vi "Create LVLIB Copies and Replace in LVPROJ.vi"(6 "copy":T1(ring), 7 "template base name":string, 8 "error in":errorcluster, 9 "CD name":string, 10 "relative path of LVLIB folders":path[](array[path]), 11 "custom device path":path) -> (0 "error out":errorcluster, 3 "custom device path out":path)   [LabVIEW 2020, in "Template Tool.lvlib"]
uses:
  Template Tool.lvlib
panel:
  out "relinked subVIs":string[](array[string])
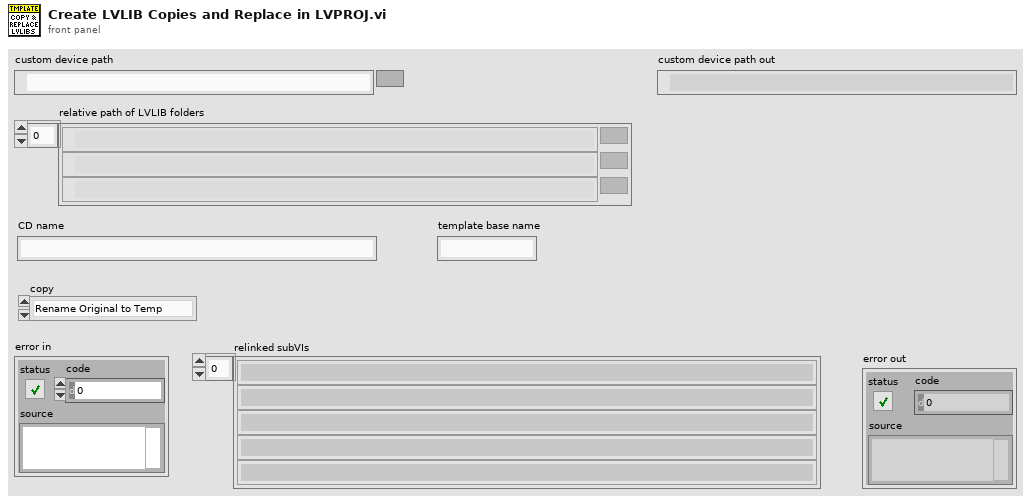
[diagram p1: front panel]
types:
  T1 = enum16{"Rename Original to Temp", "Rename Temp to Original"}
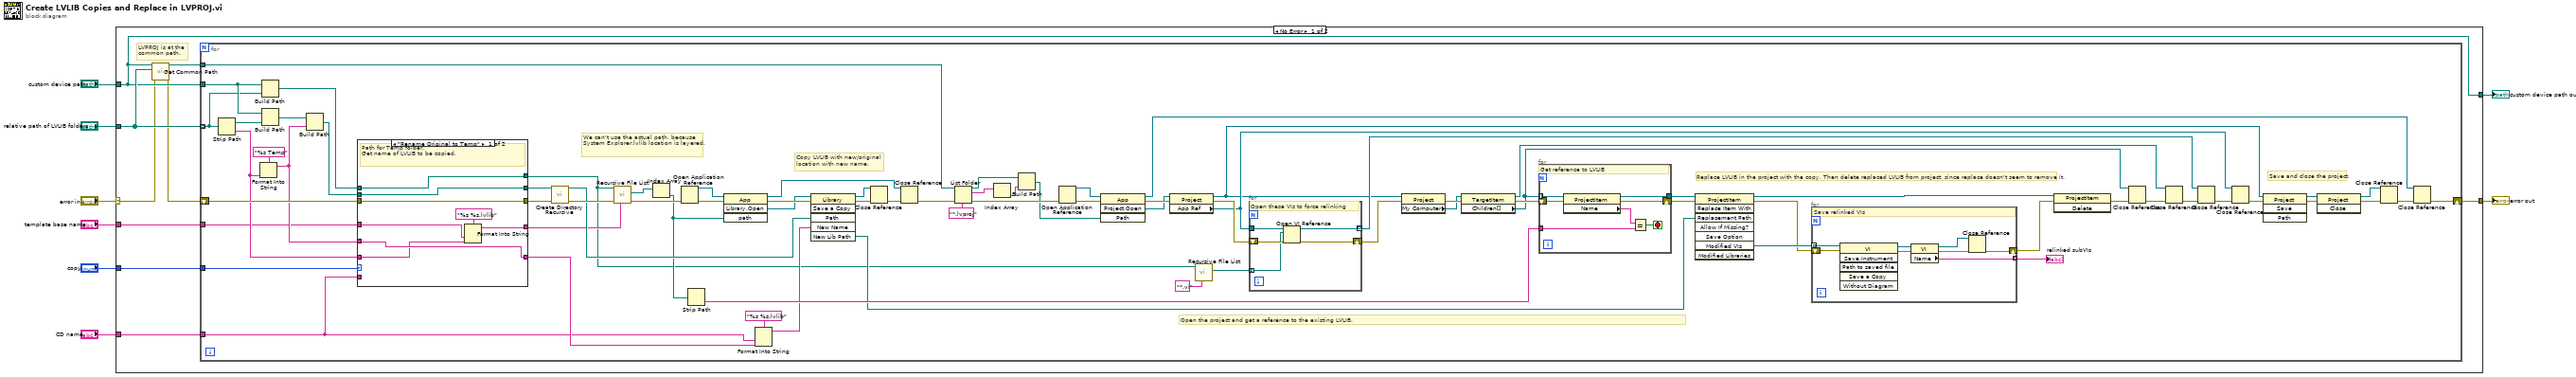
[diagram p0: block diagram]
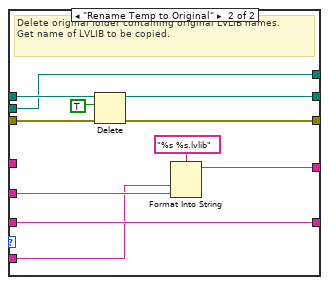
[diagram p2: hidden frame]
diagram:
  n1 = case shown="No Error" "error in" {
    selector: "error in" -> [w13 w136]
    tunnel: "custom device path" -> [w15 w135]
    tunnel: [w17 w136] -> w7
    tunnel: [w15 w135] -> w6
    tunnel: "relative path of LVLIB folders" -> [w16 _]
    tunnel: "copy" -> [w11 _]
    tunnel: "CD name" -> [w10 _]
    tunnel: "template base name" -> [w9 _]
    frame No Error {
      # "LVPROJ is at the common path."
      n2 = call "Get Common Path.vi"("error in"=w13, "relative path of LVLIB folders"=w16, "custom device path"=w15) -> ("error out"=w12:errorcluster, "common path"=w14:path)  [unwired: 7 in]
      n3 = for {
        tunnel: w15 -> [w66]
        tunnel: w16 -> [w65] mode=indexing
        shift-right: [w56] -> w17
        shift-left: w12 -> [w42]
        tunnel: w14 -> [w37]
        tunnel: w11 -> [w22]
        tunnel: w10 -> [w19]
        tunnel: w9 -> [w18]
        # "We can't use the actual path, because System Explorer.lvlib location is layered."
        # "Save and close the project."
        # "Replace LVLIB in the project with the copy. Then delete replaced LVLIB from project, since replace doesn't seem to remove it."
        # "Open the project and get a reference to the existing LVLIB."
        # "Copy LVLIB with new/original location with new name."
        n4 = Strip Path(path=w65) -> (stripped path=w67:path, name=w24:string)
        n5 = Format Into String(format string="%s Temp" ("string"), w24) -> (resulting string=w31:string)  [unwired: 2 in, 1 out]
        n6 = Build Path(base path=w66, name or relative path=w65) -> (appended path=w40:path)
        n7 = Build Path(base path=w66, name or relative path=w67) -> (appended path=w38:path)
        n8 = Build Path(base path=w38, name or relative path=w31) -> (appended path=w21:path)
        n9 = case shown="\"Rename Original to Temp\"" w22 {
          tunnel: w42 -> [w123 w133]
          tunnel: [w123 w132] -> w41
          tunnel: w40 -> [w118 w131]
          tunnel: [w122 w130] -> w39
          tunnel: [w120 w128] -> w36
          tunnel: w31 -> [w119 w127]
          tunnel: w24 -> [w117 w126]
          tunnel: [w119 w126] -> w23
          tunnel: w21 -> [w122 w125]
          tunnel: [w118 w125] -> w20
          tunnel: w19 -> [_ w124]
          tunnel: w18 -> [w116 _]
          frame "Rename Original to Temp" {
            # "Path for Temp folder.\nGet name of LVLIB to be copied."
            n10 = Format Into String(format string="%s %s.lvlib" ("pattern"), w116, w117) -> (resulting string=w120:string)  [unwired: 2 in, 1 out]
          }
          frame "Rename Temp to Original" {
            # "Delete original folder containing original LVLIB names.\nGet name of LVLIB to be copied."
            n11 = Delete(path (use dialog)=w131, entire hierarchy (F)=TRUE, error in=w133) -> (deleted path=w130:path, error out=w132:errorcluster)  [unwired: 2 in, 1 out]
            n12 = Format Into String(format string="%s %s.lvlib" ("pattern"), w124, w127) -> (resulting string=w128:string)  [unwired: 2 in, 1 out]
          }
        }
        n13 = call <vilib>:"Create Directory Recursive.vi"("error in (no error)"=w41, "directory"=w39) -> ("error out"=w87:errorcluster, "directory copy"=w53:path)  [unwired: 3 in, 1 out]
        n14 = call <vilib>:"Recursive File List.vi"("pattern"=w36, "error in (no error)"=w87, "Folder Path"=w20) -> ("error out"=w86:errorcluster, "All Files in Dir"=w95:path[])  [unwired: 4 in, 3 out]
        n15 = Index Array(array=w95) -> (element=w35:path)  [unwired: 1 in]
        n16 = Open Application Reference(8:w86) -> (0:w85:errorcluster, 3:w94:refnum<vi>)  [unwired: 3 in]
        n17 = Strip Path(path=w35) -> (name=w34:string)  [unwired: 1 out]
        n18 = invoke class="App" method="Library.Open"(reference=w94, error in=w85, "path"=w35) -> (reference out=w93:refnum<vi>, error out=w91:errorcluster, "Open Library"=w88:refnum<vi>)  [unwired: 1 in, 1 out]
        n19 = Format Into String(format string="%s %s.lvlib" ("y"), w19, w23) -> (resulting string=w29:string)  [unwired: 2 in, 1 out]
        n20 = invoke class="Library" method="Save a Copy"(reference=w88, error in=w91, "Path"=w53, "New Name"=w29) -> (reference out=w90:refnum<vi>, error out=w89:errorcluster, "New Lib Path"=w33:path)  [unwired: 2 in, 3 out]
        n21 = Close Reference(reference=w90, error in (no error)=w89) -> (error out=w92:errorcluster)
        n22 = Close Reference(reference=w93, error in (no error)=w92) -> (error out=w68:errorcluster)
        n23 = List Folder(path=w37, pattern="*.lvproj", error in=w68) -> (path out=w80:path, filenames=w79:string[], error out=w83:errorcluster)  [unwired: 1 in, 1 out]
        n24 = Index Array(array=w79) -> (element=w81:string)  [unwired: 1 in]
        n25 = Build Path(base path=w80, name or relative path=w81) -> (appended path=w64:path)
        n26 = Open Application Reference(8:w83) -> (0:w84:errorcluster, 3:w82:refnum<vi>)  [unwired: 3 in]
        n27 = invoke class="App" method="Project.Open"(reference=w82, error in=w84, "Path"=w64) -> (reference out=w71:refnum<vi>, error out=w62:errorcluster, "Project:Open"=w60:refnum<vi>)  [unwired: 1 in, 1 out]
        n28 = property class="Project"(reference=w60, error in=w62) -> (reference out=w28:refnum<vi>, error out=w63:errorcluster, "App Ref"=w58:refnum<vi>)
        n29 = call <vilib>:"Recursive File List.vi"("pattern"="*.vi", "Folder Path"=w20) -> ("All Files in Dir"=w43:path[])  [unwired: 5 in, 4 out]
        n30 = for {
          tunnel: w58 -> [w115]
          tunnel: [w112] -> w57 mode=indexing
          tunnel: w43 -> [w113] mode=indexing
          shift-right: [w111] -> w61
          shift-left: w63 -> [w114]
          # "Open these VIs to force relinking"
          n31 = Open VI Reference(application reference (local)=w115, vi path=w113, error in (no error)=w114) -> (vi reference=w112:refnum<vi>, error out=w111:errorcluster)  [unwired: 3 in]
        }
        n32 = property class="Project"(reference=w28, error in=w61) -> (error out=w76:errorcluster, "My Computer"=w75:refnum<vi>)  [unwired: 1 out]
        n33 = property class="TargetItem"(reference=w75, error in=w76) -> (reference out=w72:refnum<vi>, error out=w77:errorcluster, "Children[]"=w73:refnum<vi>[])
        n34 = for {
          tunnel: w73 -> [w110] mode=indexing
          tunnel: [w107] -> w50
          shift-right: [w105] -> w49
          shift-left: w77 -> [w106]
          tunnel: w34 -> [w104]
          stop <- w108 stop-if-true
          # "Get reference to LVLIB"
          n35 = property class="ProjectItem"(reference=w110, error in=w106) -> (reference out=w107:refnum<vi>, error out=w105:errorcluster, "Name"=w109:string)
          n36 = Equal?(x=w109, y=w104) -> (x = y?=w108:bool)
        }
        n37 = invoke class="ProjectItem" method="Replace Item With"(reference=w50, error in=w49, "Replacement Path"=w33) -> (reference out=w48:refnum<vi>, error out=w47:errorcluster, "Modified VIs"=w52:refnum<vi>[])  [unwired: 5 in, 5 out]
        n38 = for {
          tunnel: w52 -> [w101] mode=indexing
          shift-right: [w97] -> w46
          shift-left: w47 -> [w100]
          tunnel: [w99] -> w51 mode=indexing
          # "Save relinked VIs"
          n39 = invoke class="VI" method="Save.Instrument"(reference=w101, error in=w100) -> (reference out=w103:refnum<vi>, error out=w102:errorcluster)  [unwired: 4 in, 4 out]
          n40 = property class="VI"(reference=w103, error in=w102) -> (reference out=w96:refnum<vi>, error out=w98:errorcluster, "Name"=w99:string)
          n41 = Close Reference(reference=w96, error in (no error)=w98) -> (error out=w97:errorcluster)
        }
        "relinked subVIs" <- w51
        n42 = invoke class="ProjectItem" method="Delete"(reference=w48, error in=w46) -> (error out=w45:errorcluster)  [unwired: 1 in, 2 out]
        n43 = Close Reference(reference=w73, error in (no error)=w45) -> (error out=w74:errorcluster)
        n44 = Close Reference(reference=w72, error in (no error)=w74) -> (error out=w55:errorcluster)
        n45 = Close Reference(reference=w57, error in (no error)=w55) -> (error out=w59:errorcluster)
        n46 = Close Reference(reference=w58, error in (no error)=w59) -> (error out=w27:errorcluster)
        n47 = invoke class="Project" method="Save"(reference=w28, error in=w27) -> (reference out=w26:refnum<vi>, error out=w25:errorcluster)  [unwired: 2 in, 2 out]
        n48 = invoke class="Project" method="Close"(reference=w26, error in=w25) -> (reference out=w69:refnum<vi>, error out=w70:errorcluster)  [unwired: 1 in, 1 out]
        n49 = Close Reference(reference=w69, error in (no error)=w70) -> (error out=w54:errorcluster)
        n50 = Close Reference(reference=w71, error in (no error)=w54) -> (error out=w56:errorcluster)
      }
    }
    frame Error {
    }
  }
  "error out" <- w7
  "custom device path out" <- w6
